vi "export_datafile.vi"(8 "error in":errorcluster, 10 "Gains":dbl[](array[numeric])=[0.751, 0.751, 1.21], 11 "Path":path) -> (0 "error out":errorcluster, 3 "Filename":string)   [LabVIEW 2018]
uses:
  <vilib>/Utility/file.llb/Read Delimited Spreadsheet (I64).vi
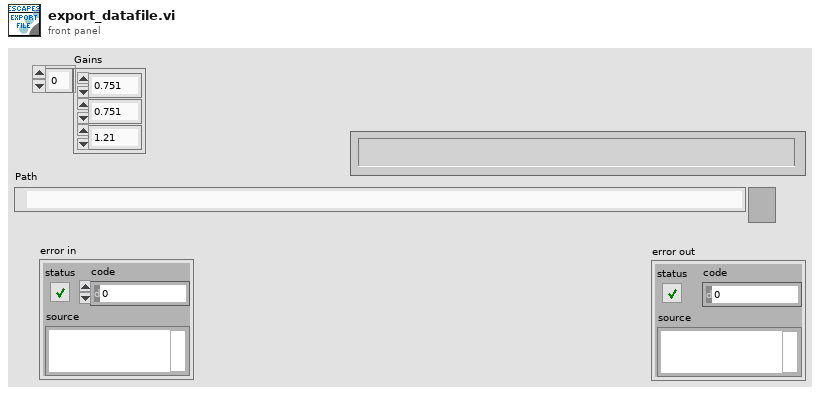
[diagram p1: front panel]
types:
  T1 = enum16{"open", "replace", "create", "open or create", "replace or create", "replace or create with confirmation"}
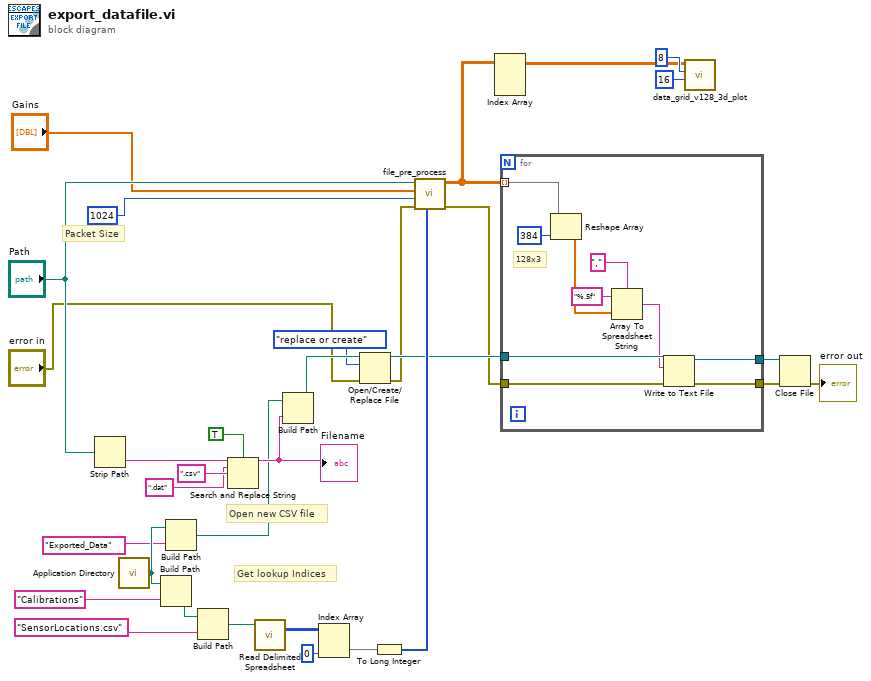
[diagram p0: block diagram]
diagram:
  # "Open new CSV file"
  # "Get lookup Indices"
  # "Packet Size"
  n1 = Strip Path(path="Path") -> (name=w21:string)  [unwired: 1 out]
  n2 = call <vilib>:"Application Directory.vi"() -> ("Application Directory"=w10:path)
  n3 = Build Path(base path=w10, name or relative path="Calibrations" ("string")) -> (appended path=w25:path)
  n4 = Build Path(base path=w10, name or relative path="Exported_Data" ("search string")) -> (appended path=w8:path)
  n5 = Build Path(base path=w25, name or relative path="SensorLocations.csv" ("string")) -> (appended path=w23:path)
  n6 = Search and Replace String(case sensitive?=TRUE ("ignore case? (F)"), input string=w21, search string=".dat", replace string=".csv" ("replace string (\"\")")) -> (result string=w17:string)  [unwired: 4 in, 3 out]
  "Filename" <- w17
  n7 = call-poly <vilib>:"Read Delimited Spreadsheet.vi"("file path (dialog if empty)"=w23) -> ("all rows"=w29:i64[][])  [unwired: 9 in, 5 out]
  n8 = Build Path(base path=w8, name or relative path=w17) -> (appended path=w18:path)
  n9 = Index Array(array=w29, index (col)=0 ("disabled index (col)")) -> (element=w27:i64[])  [unwired: 1 in]
  n10 = Open/Create/Replace File(file path (use dialog)=w18, error in="error in", operation (0:open)=T1."replace or create") -> (refnum out=w16:refnum<file>, error out=w15:errorcluster)  [unwired: 3 in, 1 out]
  n11 = To Long Integer(number=w27) -> (32bit integer=w22:i32[])
  n12 = call "file_pre_process.vi"("Sensor Lookup Indices"=w22, "error in (no error)"=w15, "Pkt Size"=i64 1024 ("count (1)"), "Gains"="Gains", "Path"="Path") -> ("error out"=w14:errorcluster, "Sensor Output - Position (mm)"=w2:dbl[][][])  [unwired: 4 in, 1 out]
  n13 = Index Array(array=w2) -> (element=w1:dbl[][])  [unwired: 3 in]
  n14 = for {
    tunnel: w2 -> [w37] mode=indexing
    tunnel: w16 -> [w42]
    tunnel: w14 -> [w41]
    tunnel: [w40] -> w12
    tunnel: [w39] -> w13
    # "128x3"
    n15 = Reshape Array(w37, 384 ("dimension size")) -> (w36:dbl[])
    n16 = Array To Spreadsheet String(delimiter (Tab)=",", array=w36, 3:"%.5f" ("format string")) -> (spreadsheet string=w38:string)
    n17 = Write to Text File(file (use dialog)=w42, text=w38, error in=w41) -> (refnum out=w39:refnum<file>, error out=w40:errorcluster)  [unwired: 1 in, 1 out]
  }
  n18 = call "data_grid_v128_3d_plot.vi"("No. Rows"=16 ("Row Length"), "No. Columns"=8, "Sensor Data"=w1) -> ()  [unwired: 6 in, 3 out]
  n19 = Close File(refnum=w13, error in=w12) -> (error out=→"error out":errorcluster)  [unwired: 1 out]
